vi "ScanNext.vi"(7 "Stage Enqueuer in":refnum<class "Message Enqueuer.lvclass">, 8 "error in":errorcluster, 9 "Scan Cluster":T2={"Scan Segments X"=0, "Scan Segments Y"=0, "X Segments Left"=0, "Y Segments Left"=0, "Acq per step"=1, "X Home"=FALSE, "Y Home"=FALSE, "Axis"=enum."X", "Acquisitions Done"=0, "Get Measurements?"=FALSE} {"Scan Segments Y" max=100 step=1 scale=0.0..100.0; "Acq per step" min=1 max=10000 step=1 scale=1.0..10000.0; "Scan Segments X" max=100 step=1 scale=0.0..100.0}, 10 "Instrument":string="KIM", 11 "MH Enqueuer in":refnum<class "Message Enqueuer.lvclass">) -> (0 "error out":errorcluster, 2 "Scan Cluster":T2={"Scan Segments X"=0, "Scan Segments Y"=0, "X Segments Left"=0, "Y Segments Left"=0, "Acq per step"=1, "X Home"=FALSE, "Y Home"=FALSE, "Axis"=enum."X", "Acquisitions Done"=0, "Get Measurements?"=FALSE} {"Scan Segments Y" max=100 step=1 scale=0.0..100.0; "Acq per step" min=1 max=10000 step=1 scale=1.0..10000.0; "Scan Segments X" max=100 step=1 scale=0.0..100.0})   [LabVIEW 2023, in "SPIController.lvlib"]
uses:
  SPIController.lvlib
  <vilib>/ActorFramework/Message Enqueuer/Message Enqueuer.lvclass
  Controller_Scan_Cluster.ctl
  SinglePhotonInterferenceUI/SinglePhotonInterferenceUI Messages/MH_Ext_Acquire Msg/MH_Ext_Acquire Msg.lvclass/MH_Ext_Acquire Msg.ctl
  <vilib>/ActorFramework/Message Enqueuer/Message Enqueuer.lvclass/Message Enqueuer.ctl
  ControllerComm/ControllerComm Mesages/AcquisitionDone Msg/AcquisitionDone Msg.lvclass/AcquisitionDone Msg.ctl
  <vilib>/ActorFramework/Message Enqueuer/Enqueue.vi
  SinglePhotonInterferenceUI/SinglePhotonInterferenceUI Messages/MH_Ext_Acquire Msg/MH_Ext_Acquire Msg.lvclass
  C:/Program Files/National Instruments/LabVIEW 2023/vi.lib/ActorFramework/Message/Message.lvclass
  ControllerComm/ControllerComm Mesages/AcquisitionDone Msg/AcquisitionDone Msg.lvclass
  SinglePhotonInterferenceUI/SinglePhotonInterferenceUI Messages/SPI_ScanDone Msg/SPI_ScanDone Msg.lvclass
  ControllerComm/ControllerComm Mesages/ScanDone Msg/ScanDone Msg.lvclass
  <vilib>/ActorFramework/Message Priority Queue/Priority Enqueue.vi
  typedefs/typedefs.lvlib
panel:
  in  "Acq Done Data":T1={"Scanning Done"=FALSE, "Axis"=enum."Y"}
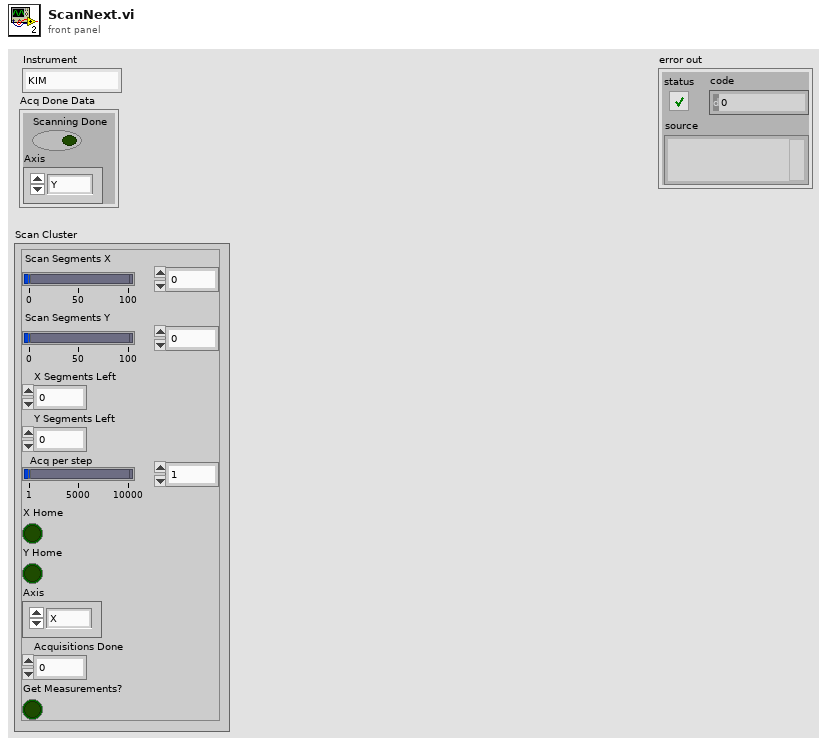
[diagram p1: front panel]
types:
  T1 = cluster{"Scanning Done":bool, "Axis":enum16{"X", "Y", "Z", "HOM"}}
  T2 = typedef "typedefs.lvlib/Controller_Scan_Cluster.ctl" = cluster{"Scan Segments X":u32, "Scan Segments Y":u32, "X Segments Left":u16, "Y Segments Left":u16, "Acq per step":u32, "X Home":bool, "Y Home":bool, "Axis":enum16{"X", "Y", "Z", "HOM"}, "Acquisitions Done":u16, "Get Measurements?":bool}
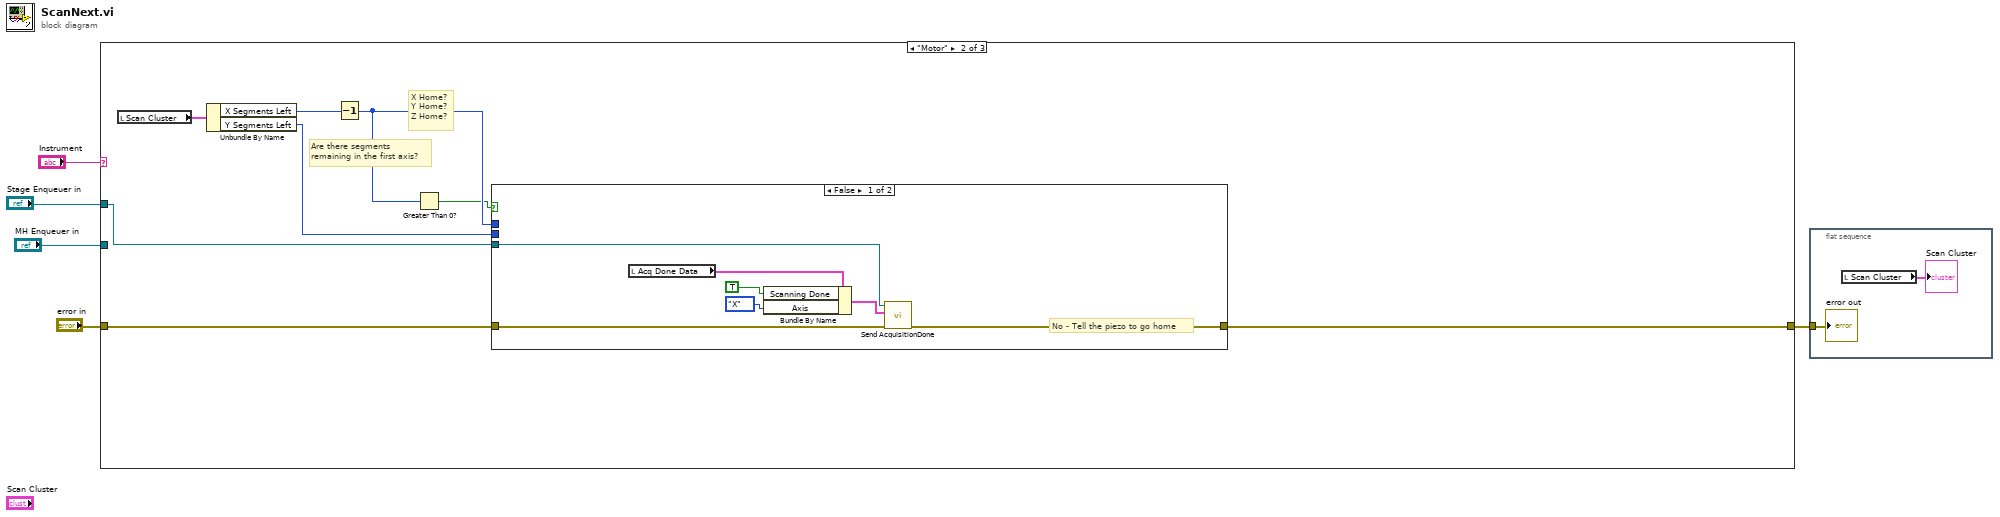
[diagram p0: block diagram]
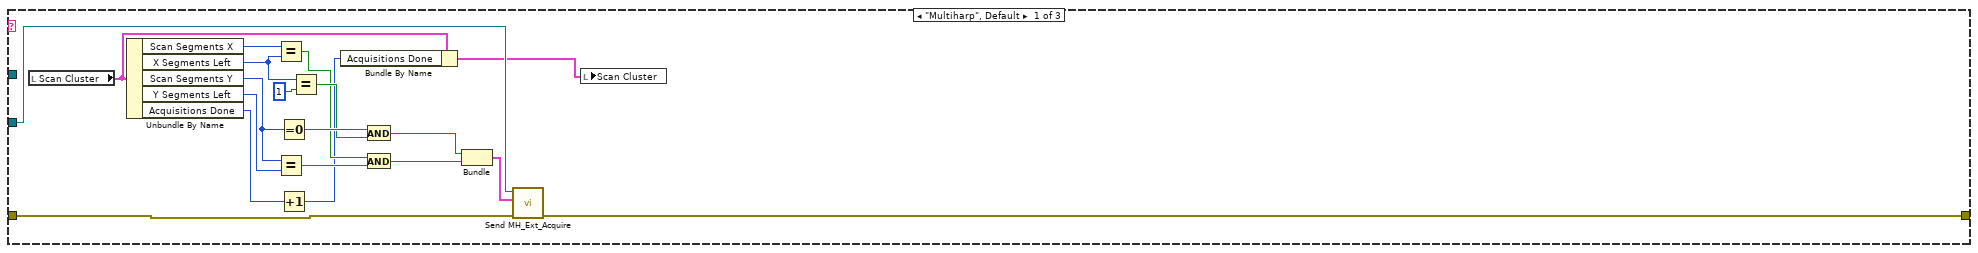
[diagram p2: hidden frame]
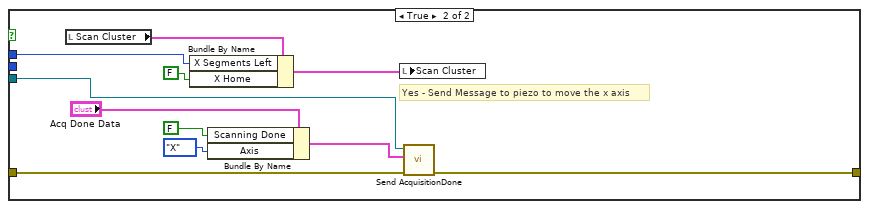
[diagram p3: hidden frame]
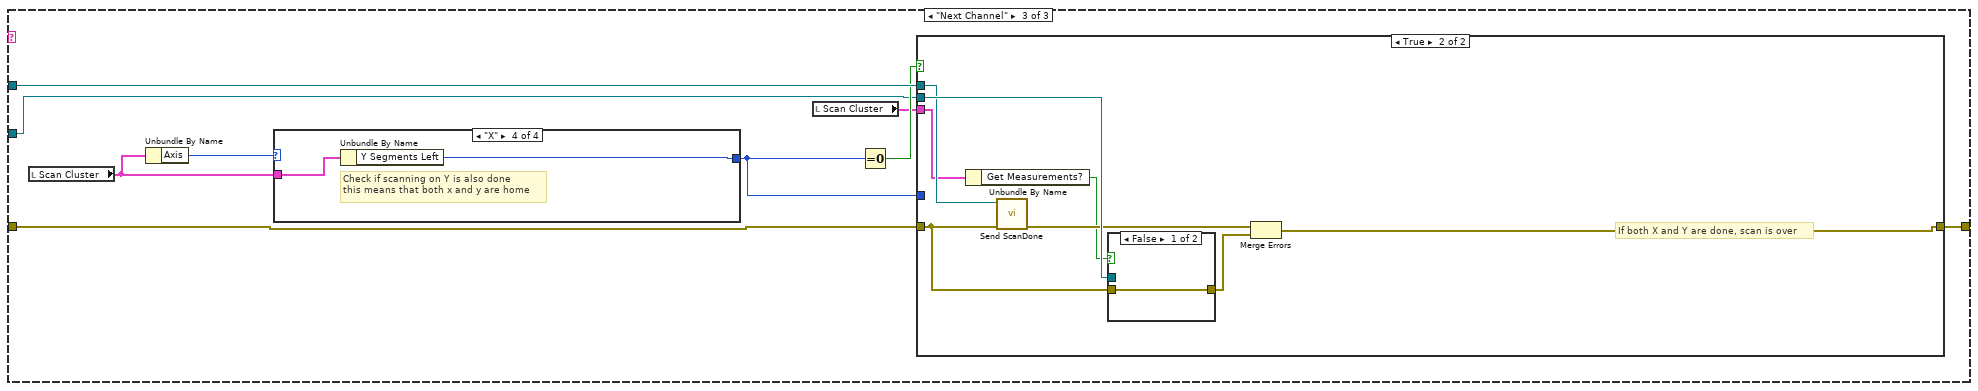
[diagram p4: hidden frame]
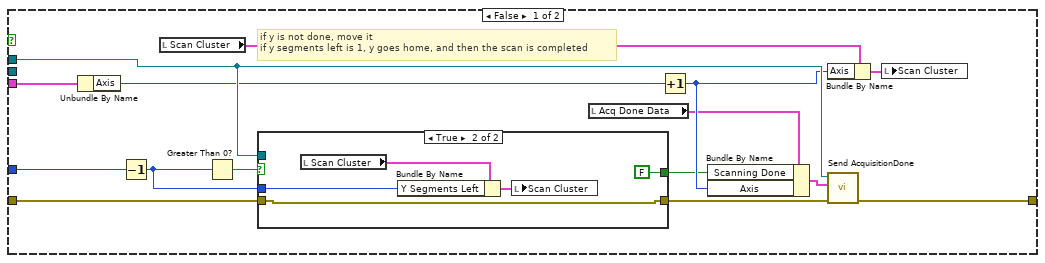
[diagram p5: hidden frame]
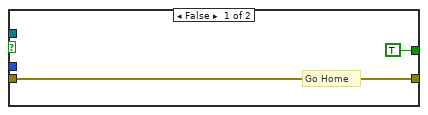
[diagram p6: hidden frame]
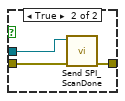
[diagram p7: hidden frame]
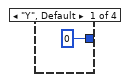
[diagram p8: hidden frame]
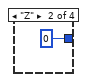
[diagram p9: hidden frame]
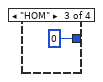
[diagram p10: hidden frame]
diagram:
  n1 = case shown="\"Motor\"" "Instrument" {
    tunnel: "MH Enqueuer in" -> [w24 _ w53]
    tunnel: "error in" -> [w22 w28 w58]
    tunnel: [w21 w29 w59] -> w4
    tunnel: "Stage Enqueuer in" -> [_ w26 w56]
    frame "Multiharp", Default {
      n2 = local read "Scan Cluster"() -> (w7:T2)
      n3 = Unbundle By Name(w7) -> ("Scan Segments X"=w20:u32, "X Segments Left"=w19:u16, "Scan Segments Y"=w14:u32, "Y Segments Left"=w13:u16, "Acquisitions Done"=w9:u16)
      n4 = Equal?(x=w20, y=w19) -> (x = y?=w11:bool)
      n5 = Equal?(x=w14, y=w13) -> (x = y?=w12:bool)
      n6 = Equal To 0?(x=w14) -> (x = 0?=w17:bool)
      n7 = Increment(x=w9) -> (x+1=w8:u16)
      n8 = Equal?(x=w19, y=u16 1) -> (x = y?=w16:bool)
      n9 = Bundle By Name(cluster=w7, "Acquisitions Done"=w8) -> (w6:T2)
      n10 = And(x=w17, y=w16) -> (x .and. y?=w15:bool)
      n11 = And(x=w11, y=w12) -> (x .and. y?=w10:bool)
      n12 = Bundle(w15, w10) -> (w23:cluster{bool, bool})  [unwired: 1 in]
      n13 = call "Send MH_Ext_Acquire.vi"("error in (no error)"=w22, "event data"=w23, "Message Enqueuer"=w24) -> ("error out"=w21:errorcluster)  [unwired: 7 in, 1 out]
      n14 = local write "Scan Cluster"(w6) -> ()
    }
    frame "Motor" {
      # "Are there segments \nremaining in the first axis?"
      # "X Home?\nY Home?\nZ Home?"
      n15 = local read "Scan Cluster"() -> (w25:T2)
      n16 = Unbundle By Name(w25) -> ("X Segments Left"=w30:u16, "Y Segments Left"=w27:u16)
      n17 = Decrement(x=w30) -> (x-1=w32:u16)
      n18 = Greater Than 0?(x=w32) -> (x > 0?=w31:bool)
      n19 = case shown="False" w31 {
        tunnel: w32 -> [_ w50]
        tunnel: w26 -> [w39 w49]
        tunnel: [w38 w48] -> w29
        tunnel: w28 -> [w37 w47]
        tunnel: w27 -> [_ _]
        frame False {
          # "No - Tell the piezo to go home"
          n20 = local read "Acq Done Data"() -> (w33:T1)
          n21 = Bundle By Name(cluster=w33, "Scanning Done"=TRUE, "Axis"=enum16{"X", "Y", "Z", "HOM"}."X") -> (w36:T1)
          n22 = call "Send AcquisitionDone.vi"("error in (no error)"=w37, "Acq Done Data"=w36, "Message Enqueuer"=w39) -> ("error out"=w38:errorcluster)  [unwired: 7 in, 1 out]
        }
        frame True {
          # "Yes - Send Message to piezo to move the x axis"
          n23 = local read "Scan Cluster"() -> (w41:T2)
          n24 = Bundle By Name(cluster=w41, "X Segments Left"=w50, "X Home"=FALSE) -> (w40:T2)
          n25 = Bundle By Name(cluster="Acq Done Data", "Scanning Done"=FALSE, "Axis"=enum16{"X", "Y", "Z", "HOM"}."X") -> (w43:T1)
          n26 = local write "Scan Cluster"(w40) -> ()
          n27 = call "Send AcquisitionDone.vi"("error in (no error)"=w47, "Acq Done Data"=w43, "Message Enqueuer"=w49) -> ("error out"=w48:errorcluster)  [unwired: 7 in, 1 out]
        }
      }
    }
    frame "Next Channel" {
      n28 = local read "Scan Cluster"() -> (w52:T2)
      n29 = Unbundle By Name(w52) -> ("Axis"=w57:enum16{"X", "Y", "Z", "HOM"})
      n30 = case shown="\"X\"" w57 {
        tunnel: [u16 0 ("Y Segments Left") u16 0 ("Y Segments Left") u16 0 ("Y Segments Left") w98] -> w55
        tunnel: w52 -> [_ _ _ w97]
        frame "Y", Default {
        }
        frame "Z" {
        }
        frame "HOM" {
        }
        frame "X" {
          # "Check if scanning on Y is also done\nthis means that both x and y are home"
          n31 = Unbundle By Name(w97) -> ("Y Segments Left"=w98:u16)
        }
      }
      n32 = local read "Scan Cluster"() -> (w51:T2)
      n33 = Equal To 0?(x=w55) -> (x = 0?=w54:bool)
      n34 = case shown="True" w54 {
        tunnel: w56 -> [w73 w86]
        tunnel: [w67 w89] -> w59
        tunnel: w58 -> [w72 w85]
        tunnel: w55 -> [w69 _]
        tunnel: w53 -> [_ w88]
        tunnel: w51 -> [w63 w82]
        frame False {
          # "if y is not done, move it\nif y segments left is 1, y goes home, and then the scan is completed"
          n35 = Unbundle By Name(w63) -> ("Axis"=w71:enum16{"X", "Y", "Z", "HOM"})
          n36 = Decrement(x=w69) -> (x-1=w68:u16)
          n37 = local read "Scan Cluster"() -> (w62:T2)
          n38 = Greater Than 0?(x=w68) -> (x > 0?=w74:bool)
          n39 = case shown="True" w74 {
            tunnel: w73 -> [_ _]
            tunnel: w72 -> [w75 w78]
            tunnel: w68 -> [_ w81]
            tunnel: [TRUE ("Scanning Done") FALSE ("Scanning Done")] -> w66
            tunnel: [w75 w78] -> w61
            frame False {
              # "Go Home"
            }
            frame True {
              n40 = local read "Scan Cluster"() -> (w79:T2)
              n41 = Bundle By Name(cluster=w79, "Y Segments Left"=w81) -> (w77:T2)
              n42 = local write "Scan Cluster"(w77) -> ()
            }
          }
          n43 = local read "Acq Done Data"() -> (w64:T1)
          n44 = Increment(x=w71) -> (x+1=w70:enum16{"X", "Y", "Z", "HOM"})
          n45 = Bundle By Name(cluster=w64, "Scanning Done"=w66, "Axis"=w70) -> (w65:T1)
          n46 = Bundle By Name(cluster=w62, "Axis"=w70) -> (w60:T2)
          n47 = call "Send AcquisitionDone.vi"("error in (no error)"=w61, "Acq Done Data"=w65, "Message Enqueuer"=w73) -> ("error out"=w67:errorcluster)  [unwired: 7 in, 1 out]
          n48 = local write "Scan Cluster"(w60) -> ()
        }
        frame True {
          # "If both X and Y are done, scan is over"
          n49 = Unbundle By Name(w82) -> ("Get Measurements?"=w83:bool)
          n50 = call "Send ScanDone.vi"("error in (no error)"=w85, "Message Enqueuer"=w86) -> ("error out"=w84:errorcluster)  [unwired: 8 in, 1 out]
          n51 = case shown="False" w83 {
            tunnel: w88 -> [_ w93]
            tunnel: w85 -> [w90 w92]
            tunnel: [w90 w91] -> w87
            frame False {
            }
            frame True {
              n52 = call "Send SPI_ScanDone.vi"("error in (no error)"=w92, "Message Enqueuer"=w93) -> ("error out"=w91:errorcluster)  [unwired: 8 in, 1 out]
            }
          }
          n53 = Merge Errors(w84, w87) -> (w89:errorcluster)
        }
      }
    }
  }
  n54 = flat-sequence {
    tunnel: w4 -> [w100]
    frame #0 {
      n55 = local read "Scan Cluster"() -> (→"Scan Cluster":T2)
      "error out" <- w100
    }
  }
